vi "VariantToProperties.vi"(0 "NHRGridSim in":refnum<class "NHRGridSim.lvclass">, 11 "error in (no error)":errorcluster) -> (4 "NHRGridSim out":refnum<class "NHRGridSim.lvclass">, 6 "Device(s)Settings":T10 {"Hardware"."Logical Instrument"."Watchdog"."Interval (s)" min=1.0 max=360.0; "Hardware"."Logical Instrument"."Safety Trips"."Pmax Sink Time (s)" min=-1.0; "Hardware"."Logical Instrument"."Safety Trips"."Pmax Sink (W)" min=0.0 format="%#_7g"; "Hardware"."Logical Instrument"."Safety Trips"."Pmax Source Time (s)" min=-1.0; "Hardware"."Logical Instrument"."Safety Trips"."Pmax Source (W)" min=0.0 format="%#_7g"; "Hardware"."Logical Instrument"."Safety Trips"."Absolute Curr Peak" min=0.0; "Hardware"."Logical Instrument"."Safety Trips"."Imax Sink Time (s)" min=-1.0; "Hardware"."Logical Instrument"."Safety Trips"."Imax Sink (A)" min=0.0; "Hardware"."Logical Instrument"."Safety Trips"."Imax Source Time (s)" min=-1.0; "Hardware"."Logical Instrument"."Safety Trips"."Imax Source (A)" min=0.0; "Hardware"."Logical Instrument"."Safety Trips"."Absolute Volt Peak" min=0.0; "Hardware"."Logical Instrument"."Safety Trips"."Vmax Time (s)" min=-1.0; "Hardware"."Logical Instrument"."Safety Trips"."Vmax (V)" min=0.0; "Hardware"."Logical Instrument"."Safety Trips"."Vmin Time (s)" min=-1.0; "Hardware"."Logical Instrument"."Safety Trips"."Vmin (V)" min=0.0; "Hardware"."Logical Instrument"."Aperture (cycles)" min=1 max=64; "Hardware"."Logical Instrument"."FreqOut (Hz)" min=0.0 max=100.0; "Hardware"."Logical Instrument"."Slew Rates"."Phase Angle Min (Deg/s)" min=0.0; "Hardware"."Logical Instrument"."Slew Rates"."Phase Angle Max (Deg/s)" min=0.0; "Hardware"."Logical Instrument"."Slew Rates"."Freq Min (Hz/s)" min=0.0; "Hardware"."Logical Instrument"."Slew Rates"."Freq Max (Hz/s)" min=0.0; "Hardware"."Logical Instrument"."Slew Rates"."Pmax (W/s)" min=0.0; "Hardware"."Logical Instrument"."Slew Rates"."Pmin (W/s)" min=0.0; "Hardware"."Logical Instrument"."Slew Rates"."Imax (A/s)" min=0.0; "Hardware"."Logical Instrument"."Slew Rates"."Vmax (V/s)" min=0.0; "Hardware"."Logical Instrument"."Slew Rates"."Imin (A/s)" min=0.0; "Hardware"."Logical Instrument"."Slew Rates"."Vmin (V/s)" min=0.0; "Hardware"."Logical Instrument"."Phases"."Change at (Deg)" min=0.0; "Hardware"."Logical Instrument"."Phases"."C-Angle (Deg)" min=0.0; "Hardware"."Logical Instrument"."Phases"."B-Angle (Deg)" min=0.0; "Hardware"."Logical Instrument"."Phases"."C-Volts (V)" min=0.0; "Hardware"."Logical Instrument"."Phases"."B-Volts (V)" min=0.0; "Hardware"."Logical Instrument"."Phases"."A-Volts (V)" min=0.0; "Hardware"."Logical Instrument"."Vout (V)" min=0.0; "Hardware"."Mode" items=["3-Phase AC"=0, "AC"=1, "DC"=2, "AC - AC"=7, "AC - DC"=8, "DC - AC"=11, "DC - DC"=12, "2-Phase AC - AC"=5, "2-Phase AC - DC"=6, "AC - AC - AC"=3, "DC - DC - DC"=4, "AC - AC - DC"=9, "AC - DC - DC"=10, "AC - DC - AC"=13, "DC - AC - AC"=14, "DC - AC - DC"=15]}, 8 "Measurements":T11 {"Instrument Number" items=["1", "2", "3"]}, 10 "MeasName":string, 13 "Measurement Refresh Time (ms)":u32, 15 "error out":errorcluster)   [LabVIEW 2018, in "AcPwrPlugins.lvlib" / "NHRGridSim.lvclass"]
doc: "This VI exposes the Device Settings, Measurement Refresh Time, Measurement Settings, and Modules properties from the variant that they were stored in."
uses:
  NHRGridSim.lvclass
  Measurements.ctl
  TypeDefs/MeasurementType.ctl
  TypeDefs/NHRGrid_Modes.ctl
  TypeDefs/NHRGrid_Phases.ctl
  TypeDefs/NHRGrid_SlewRates.ctl
  TypeDefs/NHRGrid_SafetyTrips.ctl
  TypeDefs/NHRGrid_Logical_Instrument.ctl
  TypeDefs/NHRGrid_Hardware.ctl
  TypeDefs/NHRGrid_Device(s)Settings.ctl
  TypeDefs/NHRGrid_Watchdog.ctl
  TypeDefs/NHRGrid_Ranges.ctl
  TypeDefs/NHRGrid_InstrumentCluster.ctl
panel:
  out "Hardware":T1 {"Logical Instrument"."Watchdog"."Interval (s)" min=1.0 max=360.0; "Logical Instrument"."Safety Trips"."Pmax Sink Time (s)" min=-1.0; "Logical Instrument"."Safety Trips"."Pmax Sink (W)" min=0.0 format="%#_7g"; "Logical Instrument"."Safety Trips"."Pmax Source Time (s)" min=-1.0; "Logical Instrument"."Safety Trips"."Pmax Source (W)" min=0.0 format="%#_7g"; "Logical Instrument"."Safety Trips"."Absolute Curr Peak" min=0.0; "Logical Instrument"."Safety Trips"."Imax Sink Time (s)" min=-1.0; "Logical Instrument"."Safety Trips"."Imax Sink (A)" min=0.0; "Logical Instrument"."Safety Trips"."Imax Source Time (s)" min=-1.0; "Logical Instrument"."Safety Trips"."Imax Source (A)" min=0.0; "Logical Instrument"."Safety Trips"."Absolute Volt Peak" min=0.0; "Logical Instrument"."Safety Trips"."Vmax Time (s)" min=-1.0; "Logical Instrument"."Safety Trips"."Vmax (V)" min=0.0; "Logical Instrument"."Safety Trips"."Vmin Time (s)" min=-1.0; "Logical Instrument"."Safety Trips"."Vmin (V)" min=0.0; "Logical Instrument"."Aperture (cycles)" min=1 max=64; "Logical Instrument"."FreqOut (Hz)" min=0.0 max=100.0; "Logical Instrument"."Slew Rates"."Phase Angle Min (Deg/s)" min=0.0; "Logical Instrument"."Slew Rates"."Phase Angle Max (Deg/s)" min=0.0; "Logical Instrument"."Slew Rates"."Freq Min (Hz/s)" min=0.0; "Logical Instrument"."Slew Rates"."Freq Max (Hz/s)" min=0.0; "Logical Instrument"."Slew Rates"."Pmax (W/s)" min=0.0; "Logical Instrument"."Slew Rates"."Pmin (W/s)" min=0.0; "Logical Instrument"."Slew Rates"."Imax (A/s)" min=0.0; "Logical Instrument"."Slew Rates"."Vmax (V/s)" min=0.0; "Logical Instrument"."Slew Rates"."Imin (A/s)" min=0.0; "Logical Instrument"."Slew Rates"."Vmin (V/s)" min=0.0; "Logical Instrument"."Phases"."Change at (Deg)" min=0.0; "Logical Instrument"."Phases"."C-Angle (Deg)" min=0.0; "Logical Instrument"."Phases"."B-Angle (Deg)" min=0.0; "Logical Instrument"."Phases"."C-Volts (V)" min=0.0; "Logical Instrument"."Phases"."B-Volts (V)" min=0.0; "Logical Instrument"."Phases"."A-Volts (V)" min=0.0; "Logical Instrument"."Vout (V)" min=0.0; "Mode" items=["3-Phase AC"=0, "AC"=1, "DC"=2, "AC - AC"=7, "AC - DC"=8, "DC - AC"=11, "DC - DC"=12, "2-Phase AC - AC"=5, "2-Phase AC - DC"=6, "AC - AC - AC"=3, "DC - DC - DC"=4, "AC - AC - DC"=9, "AC - DC - DC"=10, "AC - DC - AC"=13, "DC - AC - AC"=14, "DC - AC - DC"=15]}
  # "Voltages (L-N)"
  # "Voltages (L-N)"
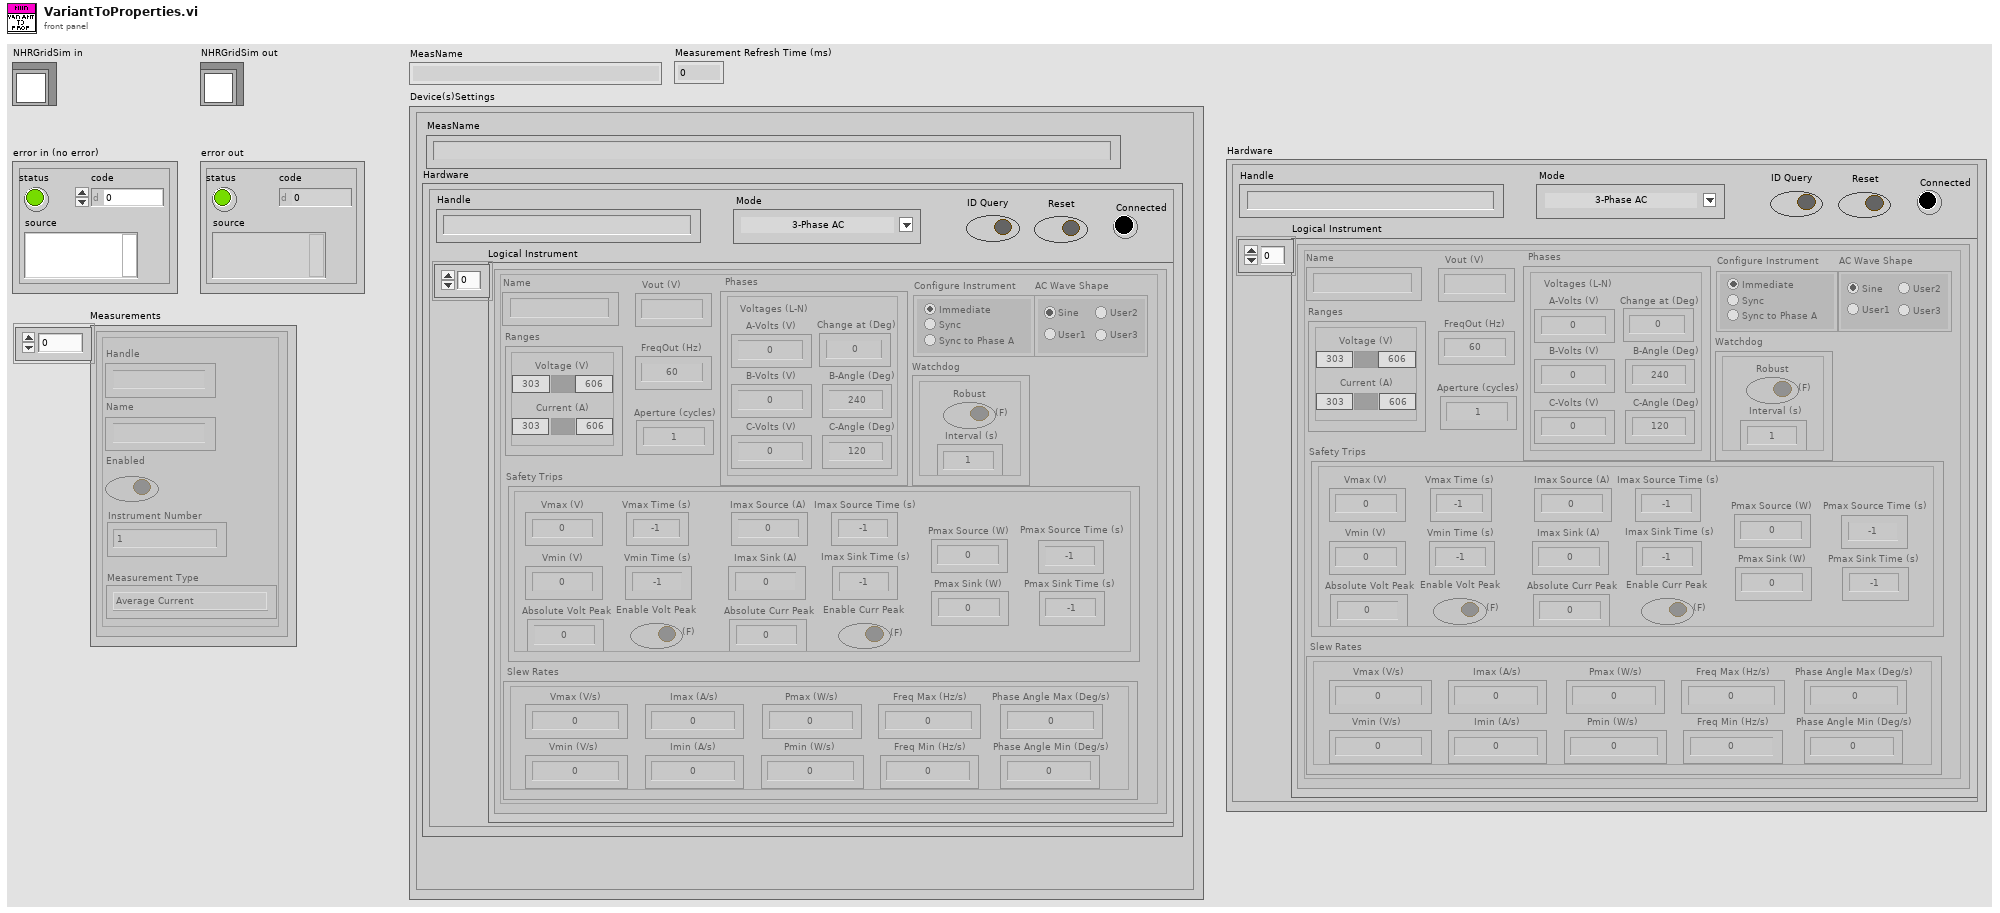
[diagram p1: front panel]
types:
  T1 = typedef "AcPwrPlugins.lvlib/NHRGridSim.lvclass/NHRGrid_Hardware.ctl" = cluster{"Handle":string, "Reset":bool, "Mode":T2, "ID Query":bool, "Connected":bool, "Logical Instrument":T3}
  T2 = typedef "AcPwrPlugins.lvlib/NHRGridSim.lvclass/NHRGrid_Modes.ctl" = u8
  T3 = typedef "AcPwrPlugins.lvlib/NHRGridSim.lvclass/NHRGrid_Logical_Instrument.ctl" = T4[]
  T4 = typedef "AcPwrPlugins.lvlib/NHRGridSim.lvclass/NHRGrid_InstrumentCluster.ctl" = cluster{"Name":string, "Vout (V)":dbl, "VType":string, "Phases":T5, "Slew Rates":T6, "FreqOut (Hz)":dbl, "Aperture (cycles)":i32, "Configure Instrument":enum32{"Conf1", "Conf2", "Conf3"}, "AC Wave Shape":enum32{"Sine", "User1", "User2", "User3"}, "Ranges":T7, "Safety Trips":T8, "Watchdog":T9}
  T5 = typedef "AcPwrPlugins.lvlib/NHRGridSim.lvclass/NHRGrid_Phases.ctl" = cluster{"A-Volts (V)":dbl, "B-Volts (V)":dbl, "C-Volts (V)":dbl, "Change at (Deg)":dbl, "B-Angle (Deg)":dbl, "C-Angle (Deg)":dbl}
  T6 = typedef "AcPwrPlugins.lvlib/NHRGridSim.lvclass/NHRGrid_SlewRates.ctl" = cluster{"Vmax (V/s)":dbl, "Vmin (V/s)":dbl, "Imax (A/s)":dbl, "Imin (A/s)":dbl, "Pmax (W/s)":dbl, "Pmin (W/s)":dbl, "Freq Max (Hz/s)":dbl, "Freq Min (Hz/s)":dbl, "Phase Angle Max (Deg/s)":dbl, "Phase Angle Min (Deg/s)":dbl}
  T7 = typedef "AcPwrPlugins.lvlib/NHRGridSim.lvclass/NHRGrid_Ranges.ctl" = cluster{"Voltage (V)":bool, "VHi":dbl, "Current (A)":bool, "CLo":dbl, "CHi":dbl, "VLo":dbl}
  T8 = typedef "AcPwrPlugins.lvlib/NHRGridSim.lvclass/NHRGrid_SafetyTrips.ctl" = cluster{"Vmax (V)":dbl, "Vmin (V)":dbl, "Vmax Time (s)":dbl, "Vmin Time (s)":dbl, "Imax Source (A)":dbl, "Imax Sink (A)":dbl, "Imax Source Time (s)":dbl, "Imax Sink Time (s)":dbl, "Pmax Source (W)":dbl, "Pmax Sink (W)":dbl, "Pmax Source Time (s)":dbl, "Pmax Sink Time (s)":dbl, "Absolute Volt Peak":dbl, "Enable Volt Peak":bool, "Absolute Curr Peak":dbl, "Enable Curr Peak":bool, "Setting t":string, "Recomm t 2":string}
  T9 = typedef "AcPwrPlugins.lvlib/NHRGridSim.lvclass/NHRGrid_Watchdog.ctl" = cluster{"Robust":bool, "Interval (s)":dbl}
  T10 = typedef "AcPwrPlugins.lvlib/NHRGridSim.lvclass/NHRGrid_Device(s)Settings.ctl" = cluster{"MeasName":string, "Hardware":T1}
  T11 = typedef "AcPwrPlugins.lvlib/NHRGridSim.lvclass/Measurements.ctl" = cluster{"Handle":string, "Name":string, "Enabled ":bool, "Measurement Value":dbl, "Instrument Number ":i32, "Measurement Type ":T12}[]
  T12 = typedef "AcPwrPlugins.lvlib/NHRGridSim.lvclass/MeasurementType.ctl" = enum16{"Average Current", "Average Voltage"}
  T13 = typedef "AcPwrPlugins.lvlib/AcPwrBase.lvclass/BaseConfig.ctl" = cluster{"Frequency":dbl, "FrequencyRange":dbl[], "Phases":T14[], "Name":string, "PluginConfigVariant":variant, "PluginMeasVariant":variant}
  T14 = typedef "AcPwrPlugins.lvlib/AcPwrBase.lvclass/Phase.ctl" = cluster{"Name":string, "Enabled":bool, "VoltageLevel":dbl, "Handle":string, "VoltageRange":dbl[], "Connected":bool, "CurrentLimit":dbl, "Waveform":string}
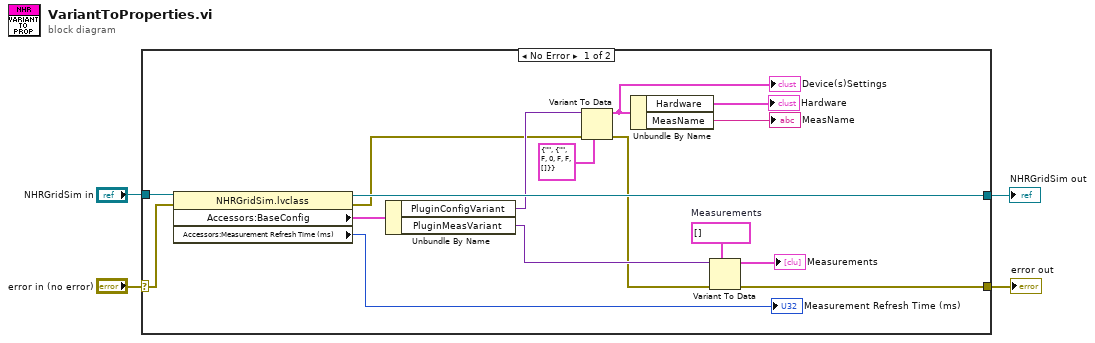
[diagram p0: block diagram]
diagram:
  n1 = case shown="No Error" "error in (no error)" {
    selector: "error in (no error)" -> [w19 w22]
    tunnel: [w5 w22] -> w1
    tunnel: "NHRGridSim in" -> [w20 w21]
    tunnel: [w18 w21] -> w2
    frame No Error {
      w16 = T11 []  # Measurements
      n2 = property class="NHRGridSim.lvclass"(reference=w20, error in=w19) -> (reference out=w18:refnum<class "NHRGridSim.lvclass">, error out=w7:errorcluster, "Accessors:BaseConfig"=w12:T13, "Accessors:Measurement Refresh Time (ms)"=→"Measurement Refresh Time (ms)":u32)
      n3 = Unbundle By Name(w12) -> ("PluginConfigVariant"=w8:variant, "PluginMeasVariant"=w17:variant)
      n4 = Variant To Data(error in=w7, type=T10 {"MeasName"="", "Hardware"={"Handle"="", "Reset"=FALSE, "Mode"=0, "ID Query"=FALSE, "Connected"=FALSE, "Logical Instrument"=[]}} ("Settings"), Variant=w8) -> (data=w13:T10, error out=w6:errorcluster)
      "Device(s)Settings" <- w13
      n5 = Unbundle By Name(w13) -> ("Hardware"=→"Hardware":T1, "MeasName"=→"MeasName":string)
      n6 = Variant To Data(error in=w6, type=w16, Variant=w17) -> (data=→"Measurements":T11, error out=w5:errorcluster)
    }
    frame Error {
    }
  }
  "error out" <- w1
  "NHRGridSim out" <- w2
